vi "Get Stages Status.vi"(8 "error in (no error)":errorcluster, 9 "XPS error in (no error)":errorcluster, 10 "Group Name (250 c max)":string, 11 "connection ID in":T1) -> (0 "error out":errorcluster, 1 "XPS error out":errorcluster, 2 "Group Status String":string, 3 "connection ID out":T1, 7 "Status":i32)   [LabVIEW 2016]
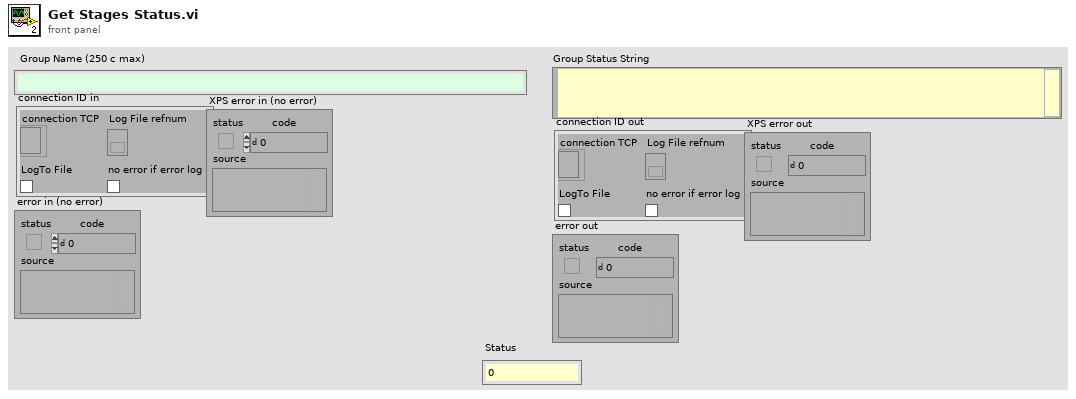
[diagram p1: front panel]
types:
  T1 = cluster{"connection TCP":refnum<k5>, "LogTo File":bool, "Log File refnum":refnum<file>, "no error if error log":bool}
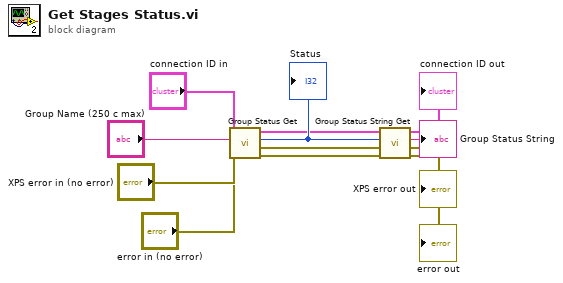
[diagram p0: block diagram]
diagram:
  n1 = call <userlib>:"Group Status Get.vi"("error in (no error)"="error in (no error)", "XPS error in (no error)"="XPS error in (no error)", "Group Name (250 c max)"="Group Name (250 c max)", "connection ID in"="connection ID in") -> ("error out"=w10:errorcluster, "XPS error out"=w11:errorcluster, "Status"=w12:i32, "connection ID out"=w9:T1)  [unwired: 4 in]
  "Status" <- w12
  n2 = call <userlib>:"Group Status String Get.vi"("error in (no error)"=w10, "XPS error in (no error)"=w11, "Status #"=w12, "connection ID in"=w9) -> ("error out"=→"error out":errorcluster, "XPS error out"=→"XPS error out":errorcluster, "Group Status String"=→"Group Status String":string, "connection ID out"=→"connection ID out":T1)  [unwired: 4 in]
